vi "OverlayMultipleLines.vi"(4 "Width":u32=1, 5 "Color":u32(colorbox)=16711680, 6 "Maintain Width?":bool, 7 "GroupName":string, 8 "error in":errorcluster, 9 "Drawing Mode (Frame)":T1, 10 "Points":T2[](array[typedef]), 11 "Image Reference In":T3) -> (0 "error out":errorcluster, 3 "Image Reference Out":T3)   [LabVIEW 2024, in "OpenLvVision_Overlays.lvlib"]
doc: "Overlaymultiple lines on top of an image."
uses:
  OpenLvVision_Overlays.lvlib
  <vilib>/OpenLvVision/OpenLvVision_Image/Management/TypeDef/OLV Image.ctl
  TypeDefs/PointI32.ctl
  TypeDefs/DrawingMode.ctl
  <vilib>/OpenLvVision/OpenLvVision_Image/Management/OLV Management.lvlib
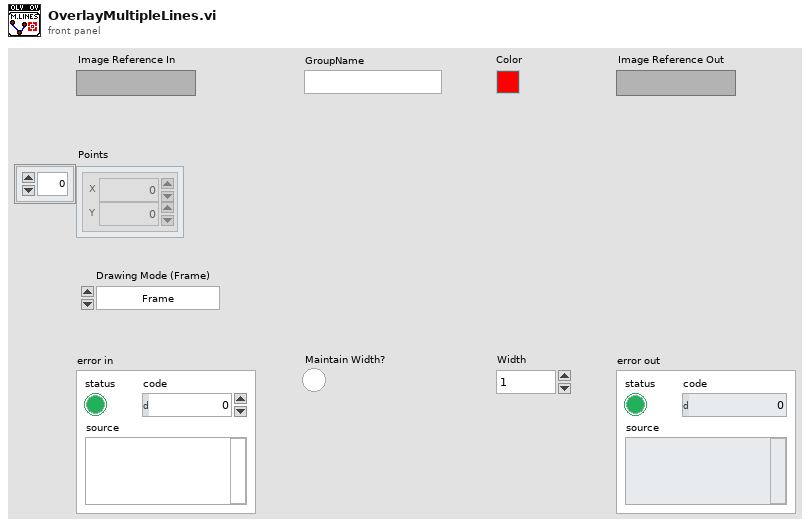
[diagram p1: front panel]
types:
  T1 = typedef "OpenLvVision_Overlays.lvlib/DrawingMode.ctl" = enum16{"Frame", "Fill"}
  T2 = typedef "OpenLvVision_Overlays.lvlib/PointI32.ctl" = cluster{"X":i32, "Y":i32}
  T3 = typedef "OLV OpenLvVision_Image.lvlib/OLV Management.lvlib/OLV Image.ctl" = refnum<image>
  T4 = typedef "IMAQ Image.ctl" = refnum<image>
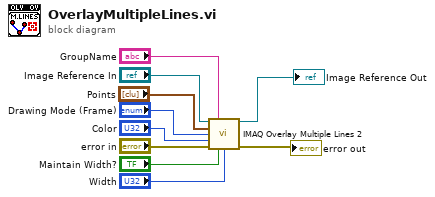
[diagram p0: block diagram]
diagram:
  n1 = call "IMAQ Overlay Multiple Lines 2"("Image"="Image Reference In", "Group"="GroupName", "Line End Points"="Points", "Drawing Mode (Frame)"="Drawing Mode (Frame)", "Color"="Color", "error in (no error)"="error in", "Maintain Width?"="Maintain Width?", "Width"="Width") -> ("Image Out"=→"Image Reference Out":T4, "error out"=→"error out":errorcluster)  [unwired: 6 in]
